vi "Script_Create Mecanum Wheel.vi"(6 "error source terminal refnum":refnum<vi>, 8 "error in (no error)":errorcluster, 10 "owner diagram refnum":refnum<vi>, 11 "wheel in":refnum<class "NI_Robotics_Wheel.lvclass">) -> (0 "error out":errorcluster, 1 "created?":bool, 2 "wheel out terminal refnum":refnum<vi>, 4 "error out terminal refnum":refnum<vi>)   [LabVIEW 2017, in "NI_Robotics_Scripting Utilities.lvlib"]
uses:
  <vilib>/robotics/Utilities/Scripting/NI_Robotics_Scripting Utilities.lvlib
  <vilib>/robotics/Steering/Wheel/NI_Robotics_Wheel.lvclass
  <vilib>/Utility/miscctls.llb/LVPointTypeDef.ctl
  <vilib>/robotics/Steering/Mecanum Wheel/Create Mecanum Wheel.vi
  <vilib>/robotics/Steering/Mecanum Wheel/NI_Robotics_Mecanum Wheel.lvclass
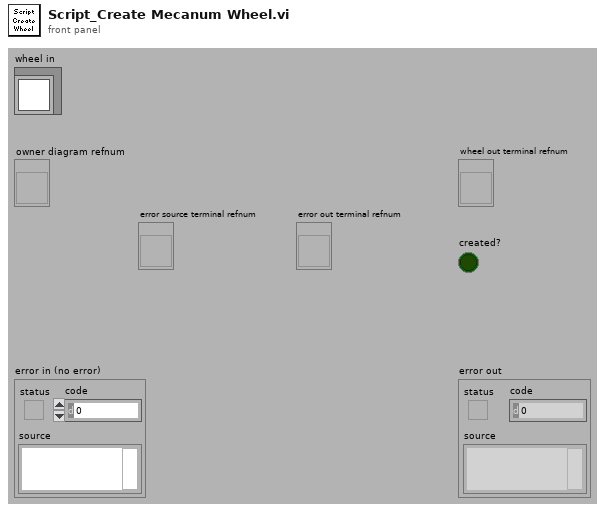
[diagram p1: front panel]
types:
  T1 = typedef "LVPointTypeDef.ctl" = cluster{"Horizontal":i16, "Vertical":i16}
  T2 = typedef "NI_Robotics_Wheel.lvclass/Wheel Parameters.ctl" = cluster{"wheel radius":dbl, "gear ratio":dbl, "forward rotation direction":T3}
  T3 = typedef "NI_Robotics_Wheel.lvclass/Rotation Direction.ctl" = u16
  T4 = typedef "NI_Robotics_Mecanum Wheel.lvclass/Roller Orientation.ctl" = u16
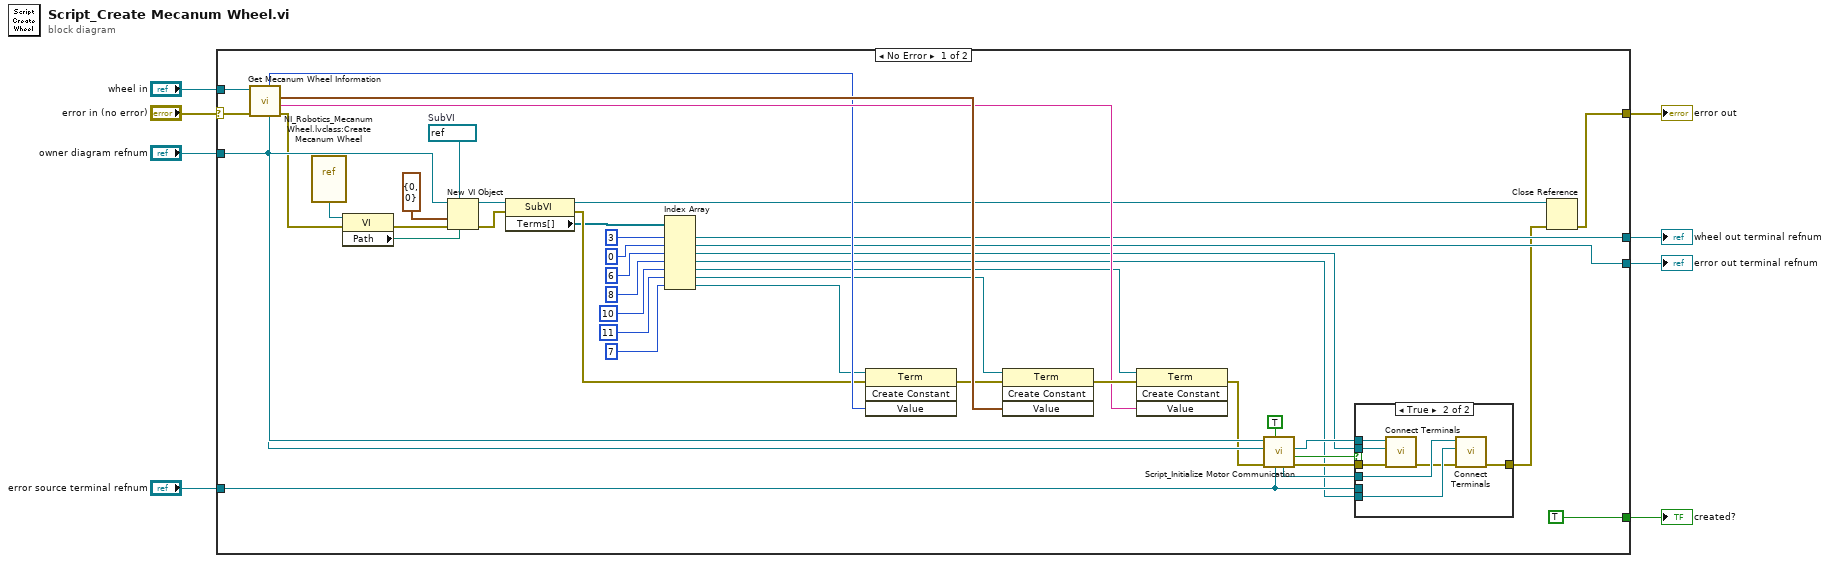
[diagram p0: block diagram]
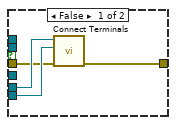
[diagram p2: hidden frame]
diagram:
  n1 = case shown="No Error" "error in (no error)" {
    selector: "error in (no error)" -> [w51 w64]
    tunnel: "wheel in" -> [w52 _]
    tunnel: [w10 w64] -> w4
    tunnel: "owner diagram refnum" -> [w42 _]
    tunnel: [w14 _] -> w2
    tunnel: [w12 _] -> w3
    tunnel: [TRUE _] -> w1
    tunnel: "error source terminal refnum" -> [w32 _]
    frame No Error {
      w48 = refnum<vi> refnum  # SubVI
      n2 = call <vilib>:"Get Mecanum Wheel Information.vi"("error in (no error)"=w51, "wheel in"=w52) -> ("error out"=w38:errorcluster, "wheel name"=w40:string, "wheel parameters"=w41:T2, "motor communication"=w50:refnum<class "NI_Robotics_Motor Communication.lvclass">, "roller orientation"=w30:T4)  [unwired: 4 in, 1 out]
      n3 = vi-ref "NI_Robotics_Mecanum Wheel.lvclass:Create Mecanum Wheel.vi"() -> (w43:refnum<vi>)
      n4 = property class="VI"(reference=w43, error in=w38) -> (error out=w47:errorcluster, "Path"=w44:path)  [unwired: 1 out]
      n5 = New VI Object(vi object class=w48, owner refnum=w42, position/next to=T1 {"Horizontal"=0, "Vertical"=0} ("relative position/next to refnum"), 6:w44, 8:w47) -> (object refnum=w29:refnum<vi>, 0:w28:errorcluster)  [unwired: 3 in]
      n6 = property class="SubVI"(reference=w29, error in=w28) -> (reference out=w11:refnum<vi>, error out=w27:errorcluster, "Terms[]"=w26:refnum<vi>[])
      n7 = Index Array(array=w26, index #1=3 ("index"), index #2=0 ("index"), index #3=6 ("index"), index #4=8 ("index"), index #5=10 ("index"), index #6=11 ("index"), index #7=7 ("index")) -> (element #1=w12:refnum<vi>, element #2=w14:refnum<vi>, element #3=w16:refnum<vi>, element #4=w18:refnum<vi>, element #5=w20:refnum<vi>, element #6=w22:refnum<vi>, element #7=w24:refnum<vi>)
      n8 = invoke class="Term" method="Create Constant"(reference=w24, error in=w27, "Value"=w30) -> (error out=w31:errorcluster)  [unwired: 1 in, 3 out]
      n9 = invoke class="Term" method="Create Constant"(reference=w22, error in=w31, "Value"=w41) -> (error out=w45:errorcluster)  [unwired: 1 in, 3 out]
      n10 = invoke class="Term" method="Create Constant"(reference=w20, error in=w45, "Value"=w40) -> (error out=w34:errorcluster)  [unwired: 1 in, 3 out]
      n11 = call <vilib>:"Script_Initialize Motor Communication.vi"("error source terminal refnum"=w32, "skip if name is empty (F)"=TRUE, "error in (no error)"=w34, "owner diagram refnum"=w42, "motor communication in"=w50) -> ("error out"=w36:errorcluster, "created?"=w37:bool, "motor communication out terminal refnum"=w39:refnum<vi>, "error out terminal refnum"=w35:refnum<vi>)  [unwired: 2 in, 1 out]
      n12 = case shown="True" w37 {
        tunnel: w39 -> [_ w60]
        tunnel: w36 -> [w54 w63]
        tunnel: w35 -> [_ w62]
        tunnel: w18 -> [w55 w61]
        tunnel: [w53 w58] -> w9
        tunnel: w32 -> [w56 _]
        tunnel: w16 -> [_ w57]
        frame False {
          n13 = call <vilib>:"Connect Terminals.vi"("error in (no error)"=w54, "sink terminal"=w55, "source terminal"=w56) -> ("error out"=w53:errorcluster)  [unwired: 7 in, 1 out]
        }
        frame True {
          n14 = call <vilib>:"Connect Terminals.vi"("error in (no error)"=w63, "sink terminal"=w57, "source terminal"=w60) -> ("error out"=w59:errorcluster)  [unwired: 7 in, 1 out]
          n15 = call <vilib>:"Connect Terminals.vi"("error in (no error)"=w59, "sink terminal"=w61, "source terminal"=w62) -> ("error out"=w58:errorcluster)  [unwired: 7 in, 1 out]
        }
      }
      n16 = Close Reference(reference=w11, error in (no error)=w9) -> (error out=w10:errorcluster)
    }
    frame Error {
    }
  }
  "error out" <- w4
  "wheel out terminal refnum" <- w3
  "error out terminal refnum" <- w2
  "created?" <- w1
